vi "Parse.vi"(8 "error in":errorcluster, 10 "Object Dictionary":refnum<class "Dictionary.lvclass">, 11 "Info Section in":refnum<class "Info Section.lvclass">) -> (0 "error out":errorcluster, 3 "Info Section out":refnum<class "Info Section.lvclass">)   [LabVIEW 2020, in "Electronic Datasheet.lvlib" / "Info Section.lvclass"]
uses:
  Info Section.lvclass
  Object Dictionary/Dictionary.lvclass
  Info Section.lvclass/Info Section.ctl
  <vilib>/Utility/Data Type/NI_Data Type.lvlib
  OD Section/Section.lvclass
  Value/Value.lvclass
  Electronic Datasheet.lvlib
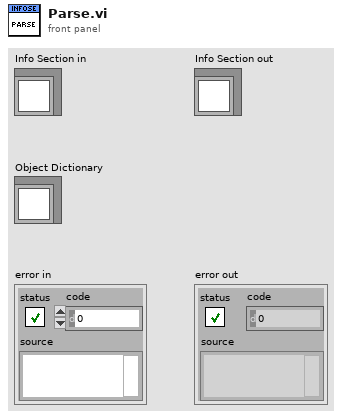
[diagram p1: front panel]
types:
  T1 = typedef "NI_Data Type.lvlib/Data Type.ctl" = enum8{"Invalid Type", "Void", "I8", "I16", "I32", "I64", "U8", "U16", "U32", "U64", "Single Float", "Double Float", "Extended Float", "Single Complex", "Double Complex", "Extended Complex", "Enum U8", "Enum U16", "Enum U32", "Enum U64", "Single Float With Unit", "Double Float With Unit", "Extended Float With Unit", "Single Complex with Unit", "Double Complex with Unit", "Extended Complex with Unit", "Boolean", "String", "Path", "Picture", "Tag", "Array", "Cluster", "Variant", "LV Variant", "Waveform", "Timestamp", "Digital Waveform", "Digital Data", "ExpressData", "Refnum", "External Data", "VI", "Poly VI", "LabVIEW Class Instance", "Fixed Point", "Set Collection", "Map Collection"}
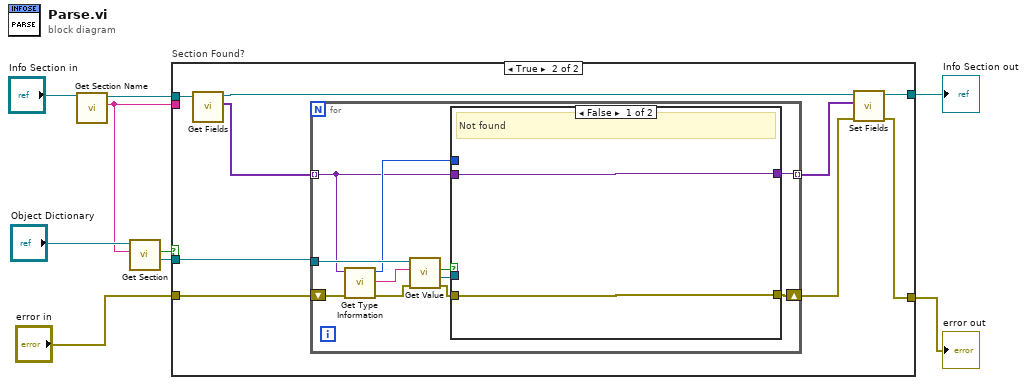
[diagram p0: block diagram]
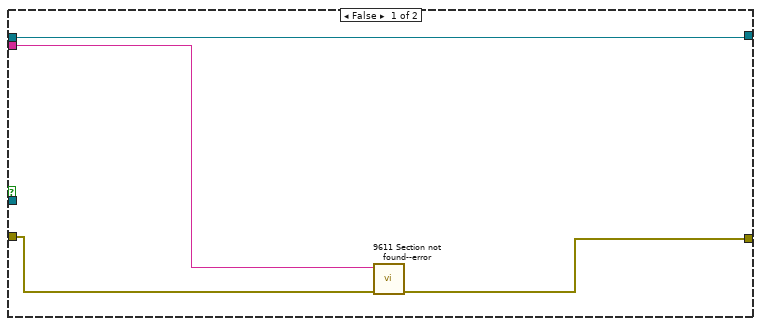
[diagram p2: hidden frame]
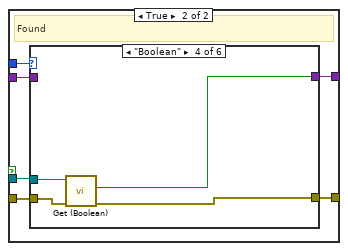
[diagram p3: hidden frame]
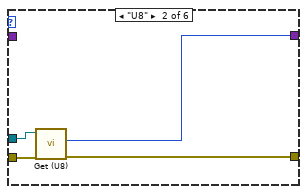
[diagram p5: hidden frame]
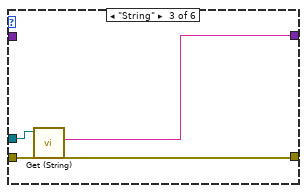
[diagram p6: hidden frame]
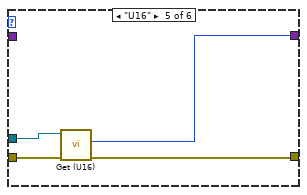
[diagram p7: hidden frame]
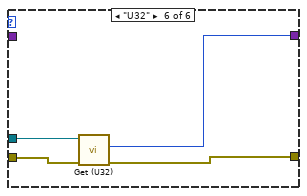
[diagram p8: hidden frame]
diagram:
  n1 = call-dynamic "Get Section Name.vi"("Info Section in"="Info Section in") -> ("Section"=w2:string, "Info Section out"=w7:refnum<class "Info Section.lvclass">)  [unwired: 9 in]
  n2 = call "Get Section.vi"("Section"=w2, "Dictionary in"="Object Dictionary") -> ("Section out"=w1:refnum<class "Section.lvclass">, "Found?"=w3:bool)  [unwired: 7 in, 1 out]
  n3 = case "Section Found?" shown="True" w3 {
    tunnel: w7 -> [w10 w22]
    tunnel: "error in" -> [w13 w21]
    tunnel: [w10 w19] -> w5
    tunnel: [w12 w17] -> w4
    tunnel: w2 -> [w11 _]
    tunnel: w1 -> [_ w14]
    frame False {
      n4 = call "9611 Section not found--error.vi"("error in"=w13, "Missing Section Name"=w11) -> ("error out"=w12:errorcluster)  [unwired: 9 in]
    }
    frame True {
      n5 = call-dynamic "Get Fields.vi"("Info Section in"=w22) -> ("Fields"=w16:variant[], "Info Section out"=w20:refnum<class "Info Section.lvclass">)  [unwired: 9 in]
      n6 = for {
        tunnel: w14 -> [w32]
        shift-right: [w28] -> w18
        shift-left: w21 -> [w33]
        tunnel: w16 -> [w23] mode=indexing
        tunnel: [w29] -> w15 mode=indexing
        n7 = call <vilib>:"Get Type Information.vi"("error in (no error)"=w33, "variant"=w23) -> ("error out"=w24:errorcluster, "name"=w30:string, "type"=w31:T1)  [unwired: 5 in, 2 out]
        n8 = call "Get Value.vi"("error in"=w24, "Key"=w30, "Section in"=w32) -> ("error out"=w27:errorcluster, "Value"=w25:refnum<class "Value.lvclass">, "Found?"=w26:bool)  [unwired: 5 in, 1 out]
        n9 = case shown="False" w26 {
          tunnel: w27 -> [w35 w41]
          tunnel: w31 -> [_ w40]
          tunnel: w25 -> [_ w39]
          tunnel: w23 -> [w34 w36]
          tunnel: [w34 w38] -> w29
          tunnel: [w35 w37] -> w28
          frame False {
            # "Not found"
          }
          frame True {
            # "Found"
            n10 = case shown="\"Boolean\"" w40 {
              tunnel: w41 -> [w42 w47 w48 w53 w56 w62]
              tunnel: [w42 w44 w48 w51 w58 w60] -> w37
              tunnel: [w43 w45 w49 w52 w55 w59] -> w38
              tunnel: w39 -> [_ w46 w50 w54 w57 w61]
              tunnel: w36 -> [w43 _ _ _ _ _]
              frame "Invalid Type", Default {
              }
              frame "U8" {
                n11 = call "Get (U8).vi"("error in"=w47, "Value in"=w46) -> ("error out"=w44:errorcluster, "Value"=w45:u8)  [unwired: 6 in, 2 out]
              }
              frame "String" {
                n12 = call "Get (String).vi"("Value in"=w50) -> ("Value"=w49:string)  [unwired: 8 in, 2 out]
              }
              frame "Boolean" {
                n13 = call "Get (Boolean).vi"("error in"=w53, "Value in"=w54) -> ("error out"=w51:errorcluster, "Value"=w52:bool)  [unwired: 6 in, 2 out]
              }
              frame "U16" {
                n14 = call "Get (U16).vi"("error in"=w56, "Value in"=w57) -> ("error out"=w58:errorcluster, "Value"=w55:u16)  [unwired: 6 in, 2 out]
              }
              frame "U32" {
                n15 = call "Get (U32).vi"("error in"=w62, "Value in"=w61) -> ("error out"=w60:errorcluster, "Value"=w59:u32)  [unwired: 6 in, 2 out]
              }
            }
          }
        }
      }
      n16 = call-dynamic "Set Fields.vi"("error in"=w18, "Fields"=w15, "Info Section in"=w20) -> ("error out"=w17:errorcluster, "Info Section out"=w19:refnum<class "Info Section.lvclass">)  [unwired: 7 in]
    }
  }
  "error out" <- w4
  "Info Section out" <- w5
